vi "Climber Check for New Command.vi"(9 "Current Command":T6, 10 "Wait time (ms)":dbl, 11 "Finished?":bool) -> (0 "Completion":T4, 1 "Subsystem Name":string, 2 "Current Command":T1, 3 "Initial Trace String":string, 4 "NextCommand":T6)   [LabVIEW 2017]
uses:
  Climber Setpoints.ctl
  Climber Operations.ctl
  <vilib>/Rock Robotics/WPI/Framework/Command Status Info.ctl
  <vilib>/Rock Robotics/WPI/Framework/Completion Status.ctl
  <vilib>/Rock Robotics/WPI/Framework/Completion Notifier.ctl
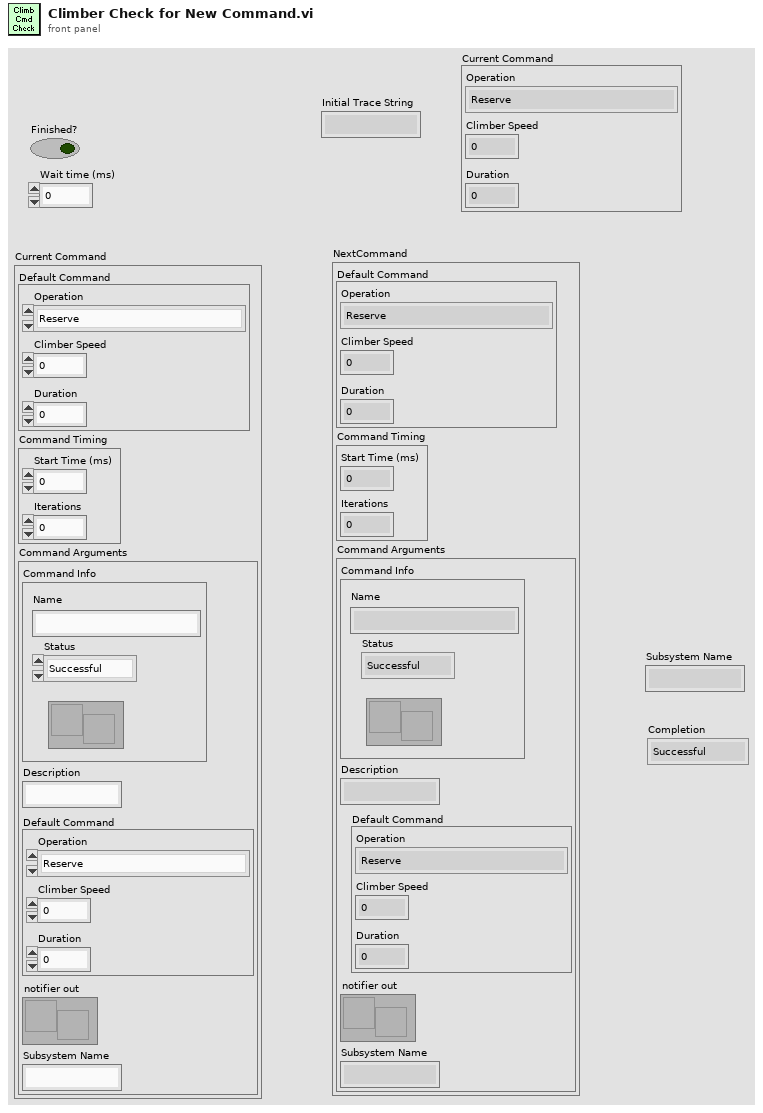
[diagram p1: front panel]
types:
  T1 = typedef "Climber Setpoints.ctl" = cluster{"Operation":T2, "Climber Speed":dbl, "Duration":dbl}
  T2 = typedef "Climber Operations.ctl" = enum16{"Reserve", "Read Current", "Climb", "Climber Out", "Climber In"}
  T3 = typedef "Command Status Info.ctl" = cluster{"Name":string, "Status":T4, "notifier out":T5}
  T4 = typedef "Completion Status.ctl" = enum16{"Successful", "Aborted", "Incomplete"}
  T5 = typedef "Completion Notifier.ctl" = refnum<notifier>
  T6 = cluster{"Default Command":T1, "Command Timing":cluster{"Start Time (ms)":u32, "Iterations":i32}, "Command Arguments":cluster{"Command Info":T3, "Description":string, "Default Command":T1, "notifier out":refnum<notifier>, "Subsystem Name":string}}
  T7 = cluster{"Command Info":T3, "Description":string, "Default Command":T1, "notifier out":refnum<notifier>, "Subsystem Name":string}
  T8 = cluster{"Default Command":T1, "Command Info":T3, "Description":string}
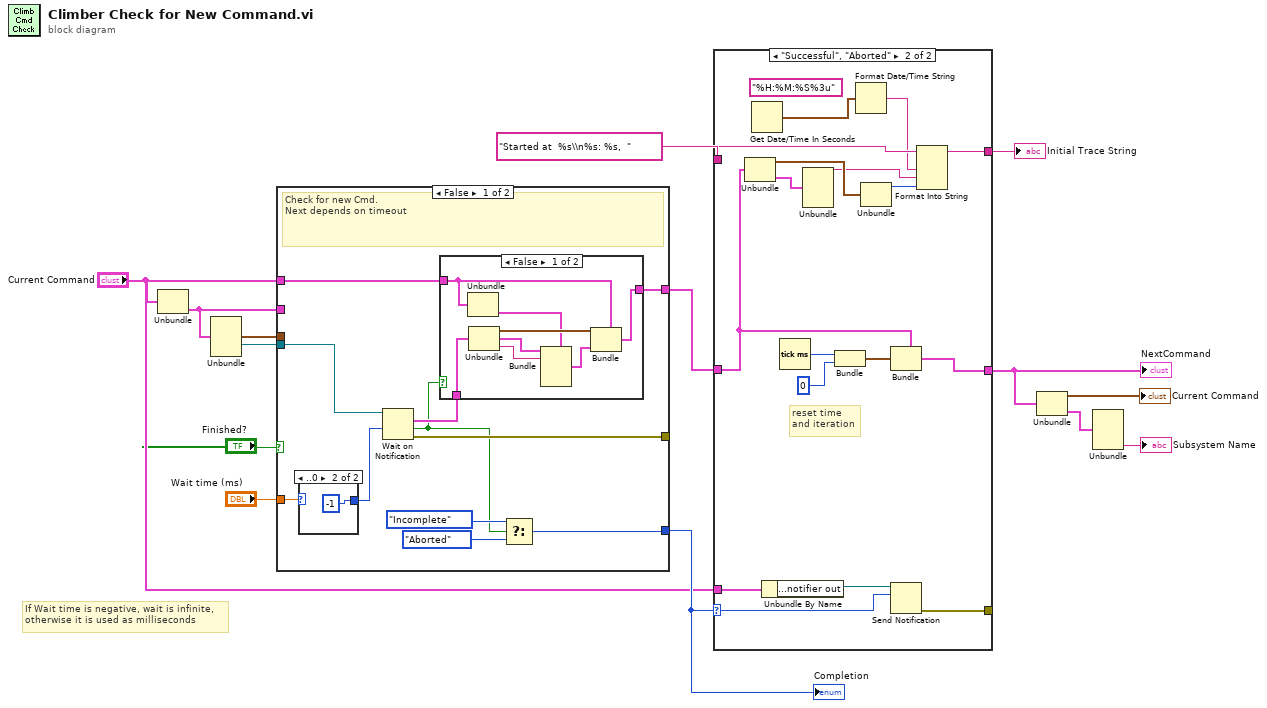
[diagram p0: block diagram]
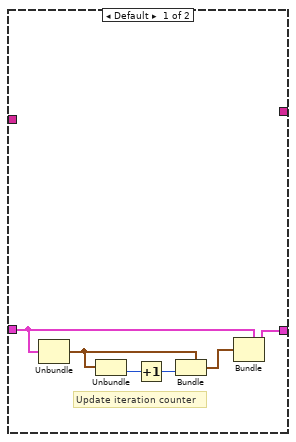
[diagram p2: hidden frame]
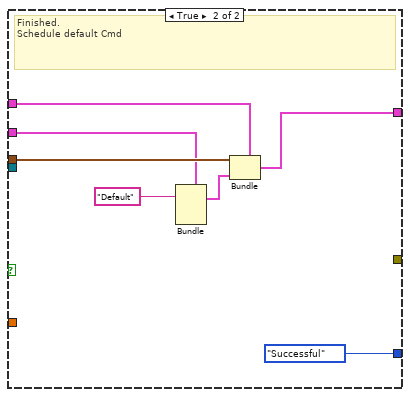
[diagram p5: hidden frame]
diagram:
  # "If Wait time is negative, wait is infinite,\notherwise it is used as milliseconds"
  n1 = Unbundle("Current Command") -> ("Command Arguments"=w1:T7)  [unwired: 2 out]
  n2 = Unbundle(w1) -> ("Default Command"=w4:T1, "notifier out"=w5:refnum<notifier>)  [unwired: 3 out]
  n3 = case shown="False" "Finished?" {
    tunnel: [w15 w42] -> w10
    tunnel: "Wait time (ms)" -> [w20 _]
    tunnel: [w23 Completion_Status."Successful"] -> w14
    tunnel: [w25 _] -> _
    tunnel: w5 -> [w24 _]
    tunnel: "Current Command" -> [w17 w41]
    tunnel: w4 -> [_ w40]
    tunnel: w1 -> [_ w38]
    frame False {
      # "Check for new Cmd.\nNext depends on timeout"
      n4 = case shown="..0" w20 {
        selector: w20 -> [w35 _]
        tunnel: [w35 -1] -> w19
        frame Default {
        }
        frame ..0 {
        }
      }
      n5 = Wait on Notification(notifier=w24, timeout in ms (-1)=w19) -> (notification=w18:T8, timed out?=w16:bool, error out=w25:errorcluster)  [unwired: 2 in, 1 out]
      n6 = case shown="False" w16 {
        tunnel: w18 -> [w33 _]
        tunnel: w17 -> [w30 w34]
        tunnel: [w26 w34] -> w15
        frame False {
          n7 = Unbundle(w30) -> ("Command Arguments"=w29:T7)  [unwired: 2 out]
          n8 = Unbundle(w33) -> ("Default Command"=w32:T1, "Command Info"=w27:T3, "Description"=w28:string)
          n9 = Bundle(cluster=w29, "Command Info"=w27, "Description"=w28) -> (w31:T7)  [unwired: 3 in]
          n10 = Bundle(cluster=w30, "Default Command"=w32, "Command Arguments"=w31) -> (w26:T6)  [unwired: 1 in]
        }
        frame True {
        }
      }
      n11 = Select(t=Completion_Status."Incomplete", s=w16, f=Completion_Status."Aborted") -> (s? t:f=w23:T4)
    }
    frame True {
      # "Finished.\nSchedule default Cmd"
      n12 = Bundle(cluster=w38, "Description"="Default") -> (w39:T7)  [unwired: 4 in]
      n13 = Bundle(cluster=w41, "Default Command"=w40, "Command Arguments"=w39) -> (w42:T6)  [unwired: 1 in]
    }
  }
  "Completion" <- w14
  n14 = case shown="\"Successful\", \"Aborted\"" w14 {
    selector: w14 -> [_ w66]
    tunnel: "Current Command" -> [_ w63]
    tunnel: "Started at  %s\\n%s: %s,  " ("format string") -> [_ w62]
    tunnel: [_ w61] -> w12
    tunnel: w10 -> [w46 w50]
    tunnel: [w47 w57] -> w9
    tunnel: [_ w54] -> _
    frame Default {
      # "Update iteration counter"
      n15 = Unbundle(w46) -> ("Command Timing"=w45:cluster{"Start Time (ms)":u32, "Iterations":i32})  [unwired: 2 out]
      n16 = Unbundle(w45) -> ("Iterations"=w48:i32)  [unwired: 1 out]
      n17 = Increment(x=w48) -> (x+1=w49:i32)
      n18 = Bundle(cluster=w45, "Iterations"=w49) -> (w44:cluster{"Start Time (ms)":u32, "Iterations":i32})  [unwired: 1 in]
      n19 = Bundle(cluster=w46, "Command Timing"=w44) -> (w47:T6)  [unwired: 2 in]
    }
    frame "Successful", "Aborted" {
      (unwired) "%H:%M:%S%3u" ("time format string (%c)")
      # "reset time\nand iteration"
      n20 = Unbundle(w50) -> ("Default Command"=w60:T1, "Command Arguments"=w55:T7)  [unwired: 1 out]
      n21 = Get Date/Time In Seconds() -> (seconds since 1Jan1904=w53:timestamp)
      n22 = Unbundle By Name(w63) -> ("Command Arguments.Command Info.notifier out"=w65:T5)
      n23 = Tick Count (ms)() -> (millisecond timer value=w59:u32)
      n24 = Unbundle(w55) -> ("Description"=w52:string)  [unwired: 4 out]
      n25 = Bundle("millisecond timer value"=w59, 0) -> (w56:cluster{"millisecond timer value":u32, i32})  [unwired: 1 in]
      n26 = Format Date/Time String(seconds (now)=w53) -> (date/time string=w51:string)  [unwired: 2 in]
      n27 = Unbundle(w60) -> ("Operation"=w64:T2)  [unwired: 2 out]
      n28 = Bundle(cluster=w50, "Command Timing"=w56) -> (w57:T6)  [unwired: 2 in]
      n29 = Send Notification(notification=w66, notifier=w65) -> (error out=w54:errorcluster)  [unwired: 1 in, 1 out]
      n30 = Format Into String(format string=w62, w51, w52, w64) -> (resulting string=w61:string)  [unwired: 2 in, 1 out]
    }
  }
  "NextCommand" <- w9
  "Initial Trace String" <- w12
  n31 = Unbundle(w9) -> ("Default Command"=→"Current Command":T1, "Command Arguments"=w3:T7)  [unwired: 1 out]
  n32 = Unbundle(w3) -> ("Subsystem Name"=→"Subsystem Name":string)  [unwired: 4 out]
